vi "1820_PS_ON_duration.vi"(10 "SWITCH HEATER":bool, 11 "time stamp":timestamp format="%<%I:%M:%S %p>T") -> (3 "PS Heat on (sec)":dbl)   [LabVIEW 2016]
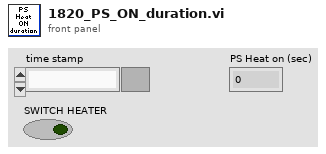
[diagram p1: front panel]
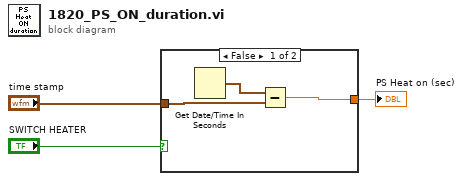
[diagram p0: block diagram]
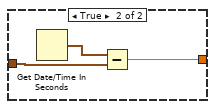
[diagram p2: hidden frame]
diagram:
  n1 = case shown="False" "SWITCH HEATER" {
    tunnel: "time stamp" -> [w5 w7]
    tunnel: [w4 w8] -> w1
    frame False {
      n2 = Get Date/Time In Seconds() -> (seconds since 1Jan1904=w6:timestamp)
      n3 = Subtract(x=w6, y=w5) -> (x-y=w4:dbl)
    }
    frame True {
      n4 = Get Date/Time In Seconds() -> (seconds since 1Jan1904=w9:timestamp)
      n5 = Subtract(x=w9, y=w7) -> (x-y=w8:dbl)
    }
  }
  "PS Heat on (sec)" <- w1
